vi "Configure Devices.vi"(8 "error in":errorcluster, 11 "Device in":refnum<class "Device.lvclass">) -> (0 "error out":errorcluster, 3 "Device out":refnum<class "Device.lvclass">)   [LabVIEW 2015, in "DAQ Device.lvlib" / "Device.lvclass"]
uses:
  Device.lvclass
  <vilib>/ActorFramework/Actor/Actor.lvclass/Actor.ctl
  Device.lvclass/Device.ctl
  DAQ Device/Cfg Msg.ctl
  <vilib>/MSR Consulting, LLC/Configurable Device/Configurable Device.lvclass/Configurable Device.ctl
  Messages/Device Configuration/Get Serialized Device Configuration MSG.lvclass/Get Serialized Device Configuration MSG.ctl
  <vilib>/ActorFramework/Message Enqueuer/Message Enqueuer.lvclass/Message Enqueuer.ctl
  Messages/Generic CVT Init/Generic Init CVT Message.lvclass/Generic Init CVT Message.ctl
  Messages/Generic CVT Init/Write DevID.vi
  Messages/Generic CVT Init/Write SP.vi
  <vilib>/MSR Consulting, LLC/Configurable Device/Read ID.vi
  <vilib>/MSR Consulting, LLC/Configurable Device/Accessors/Read Device Type.vi
  <vilib>/MSR Consulting, LLC/Configurable Device/Accessors/Read label.vi
  <vilib>/MSR Consulting, LLC/Configurable Device/Accessors/Read SN.vi
  <vilib>/MSR Consulting, LLC/Configurable Device/Read controller_.vi
  <vilib>/MSR Consulting, LLC/Configurable Device/Accessors/Read Addr.vi
  <vilib>/MSR Consulting, LLC/Configurable Device/Accessors/Read Model.vi
  <vilib>/MSR Consulting, LLC/Configurable Device/Read Device Active_.vi
  Messages/Device Configuration/Write cfg cluster.vi
  <vilib>/ActorFramework/Message Priority Queue/Priority Enqueue.vi
  <vilib>/MSR Consulting, LLC/General Reuse/SuperActor/xGlobal Data.vi
  <vilib>/MSR Consulting, LLC/Configurable Device/Configurable Device.lvclass
  <vilib>/ActorFramework/Actor/Actor.lvclass
  <vilib>/ActorFramework/Message Enqueuer/Message Enqueuer.lvclass
  DAQ Device.lvlib
  <vilib>/MSR Consulting, LLC/General Reuse/SuperActor/SuperActor.lvclass
  Messages/Generic CVT Init/Generic Init CVT Message.lvclass
  Messages/Device Configuration/Get Serialized Device Configuration MSG.lvclass
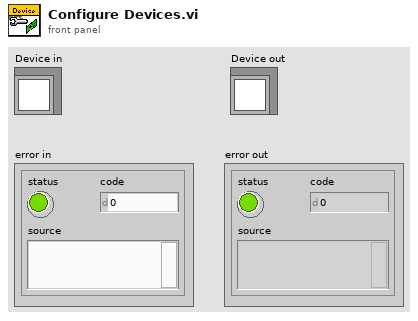
[diagram p1: front panel]
types:
  T1 = typedef "DAQ Device.lvlib/Cfg Msg.ctl" = cluster{"ID":string, "type":string, "label":string, "SN":string, "controller_":bool, "Addr":string, "Model":string, "Device Active":bool}
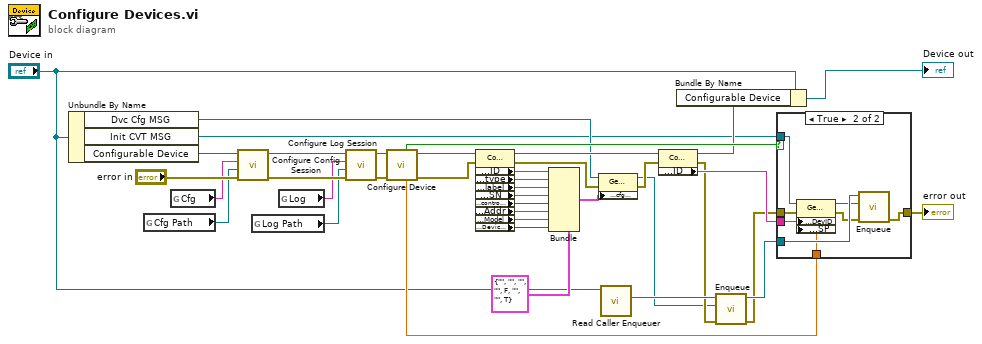
[diagram p0: block diagram]
diagram:
  n1 = Unbundle By Name("Device in") -> ("Dvc Cfg MSG"=w13:refnum<class "Get Serialized Device Configuration MSG.lvclass">, "Init CVT MSG"=w12:refnum<class "Generic Init CVT Message.lvclass">, "Configurable Device"=w11:refnum<class "Configurable Device.lvclass">)
  n2 = global read "xGlobal Data.vi" "Cfg Path"() -> (w3:path)
  n3 = global read "xGlobal Data.vi" "Cfg"() -> (w2:string)
  n4 = call <vilib>:"Configure Config Session.vi"("error in"="error in", "Path"=w3, "Ref Name"=w2, "Configurable Device in"=w11) -> ("error out"=w7:errorcluster, "Configurable Device out"=w10:refnum<class "Configurable Device.lvclass">)  [unwired: 6 in]
  n5 = global read "xGlobal Data.vi" "Log Path"() -> (w4:path)
  n6 = global read "xGlobal Data.vi" "Log"() -> (w5:string)
  n7 = call <vilib>:"Configure Log Session.vi"("error in"=w7, "Path"=w4, "Ref Name"=w5, "Configurable Device in"=w10) -> ("error out"=w6:errorcluster, "Configurable Device out"=w9:refnum<class "Configurable Device.lvclass">)  [unwired: 6 in]
  n8 = call-dynamic "Configure Device.vi"("error in"=w6, "Device in"=w9) -> ("error out"=w16:errorcluster, "Device out"=w29:refnum<class "Configurable Device.lvclass">, "SP"=w33:dbl, "Settable?"=w37:bool)  [unwired: 6 in]
  n9 = property class="Configurable Device"(reference=w29, error in=w16) -> (reference out=w18:refnum<class "Configurable Device.lvclass">, error out=w15:errorcluster, "Accessors:ID"=w28:string, "Accessors:type"=w27:string, "Accessors:label"=w26:string, "Accessors:SN"=w25:string, "Accessors:controller_"=w24:bool, "Accessors:Addr"=w23:string, "Accessors:Model"=w17:string, "Accessors:Device Active_"=w1:bool)
  n10 = Bundle(cluster=T1 {"ID"="", "type"="", "label"="", "SN"="", "controller_"=FALSE, "Addr"="", "Model"="", "Device Active"=TRUE}, "ID"=w28, "type"=w27, "label"=w26, "SN"=w25, "controller_"=w24, "Addr"=w23, "Model"=w17, "Device Active"=w1) -> (w21:T1)
  n11 = property class="Get Serialized Device Configura"(reference=w13, error in=w15, "Accessors:cfg cluster"=w21) -> (reference out=w19:refnum<class "Get Serialized Device Configuration MSG.lvclass">, error out=w20:errorcluster)
  n12 = call <vilib>:"Read Caller Enqueuer.vi"("Actor"="Device in") -> ("Caller Enqueuer"=w38:refnum<class "Message Enqueuer.lvclass">)  [unwired: 10 in]
  n13 = property class="Configurable Device"(reference=w18, error in=w20) -> (reference out=w35:refnum<class "Configurable Device.lvclass">, error out=w32:errorcluster, "Accessors:ID"=w34:string)
  n14 = Bundle By Name(cluster="Device in", "Configurable Device"=w35) -> (→"Device out":refnum<class "Device.lvclass">)
  n15 = call <vilib>:"Enqueue.vi"("error in (no error)"=w32, "Message"=w19, "Message Enqueuer in"=w38) -> ("error out"=w31:errorcluster, "Message Enqueuer out"=w36:refnum<class "Message Enqueuer.lvclass">)  [unwired: 7 in]
  n16 = case shown="True" w37 {
    tunnel: w36 -> [_ w48]
    tunnel: w12 -> [_ w47]
    tunnel: w34 -> [_ w46]
    tunnel: w33 -> [_ w45]
    tunnel: w31 -> [w40 w42]
    tunnel: [w40 w41] -> w30
    frame False {
    }
    frame True {
      n17 = property class="Generic Init CVT Message"(reference=w47, error in=w42, "Accessors:DevID"=w46, "Accessors:SP"=w45) -> (reference out=w44:refnum<class "Generic Init CVT Message.lvclass">, error out=w43:errorcluster)
      n18 = call <vilib>:"Enqueue.vi"("error in (no error)"=w43, "Message"=w44, "Message Enqueuer in"=w48) -> ("error out"=w41:errorcluster)  [unwired: 7 in, 1 out]
    }
  }
  "error out" <- w30
